vi "USRP Packet Transmitter(working).vi"(8 "Tx Parameters":T7={"Tx IQ Sampling\nRate [s/sec]"=500000.0, "Tx Frequency [Hz]"=2500000000.0, "Tx Gain [dB]"=0.0, "Tx Antenna"="TX1"} {"Tx Gain [dB]" format="%#.6p"; "Tx Frequency [Hz]" format="%#.6p"; "Tx IQ Sampling\nRate [s/sec]" format="%#.6p"}, 9 "USRP IP address":refnum<k15>="192.168.10.2", 10 "working directory":path=path "C:/perlTest") -> (1 "Constellation Graph":T1(graph), 2 "error out":errorcluster, 3 "standard output":string)   [LabVIEW 2022 SP3]
uses:
  <instrlib>/niUSRP/niUSRP Write Tx Data (CDB Cluster).vi
  <vilib>/addons/Modulation/Digital/General/MT Generate PSK System Parameters(M).vi
  <vilib>/addons/Modulation/niDMT.lvlib
panel:
  out "return value":string
  in  "module path":path
  out "error out 2":errorcluster
  in  "autoscale":bool
  out "Symbol Rate\n[symbols/sec]":dbl=25000.0 format="%#.6p"
  in  "stop":bool
  in  "Tab Control":T2(tab)
  in  "command line":string
  in  "Packet Parameters":T3={"Guard Bits "=30, "Sync Bits"=20, "Message Bits"=128}
  in  "Packet Pad \n[samples]":i32=200
  in  "Blank Frame \n[samples]":i32=500
  out "Number of Packets in Message":i32=46
  in  "PN sequence order\nfor Sync Bits":i32=31 caption="PN sequence order (9)"
  in  "Packet Repeat":i32=2
  in  "Select PSK Modulation Format":T4(tab)=enum."QPSK" caption="PSK"
  in  "BPSK System Parameters":T5={"Samples per Symbol"=8, "symbol map"=[], "Differential PSK"=enum."disable", "PSK type"=0} {"PSK type" items=["normal", "shifted", "offset"]; "symbol map" format="%.3f"}
  in  "QPSK System Parameters":T5={"Samples per Symbol"=8, "symbol map"=[], "Differential PSK"=enum."disable", "PSK type"=0} {"PSK type" items=["normal", "shifted", "offset"]; "symbol map" format="%.3f"}
  in  "pi/4 DQPSK System Parameters":T5={"Samples per Symbol"=8, "symbol map"=[], "Differential PSK"=enum."enable", "PSK type"=1} {"PSK type" items=["normal", "shifted", "offset"]; "symbol map" format="%.3f"}
  in  "OQPSK System Parameters":T5={"Samples per Symbol"=8, "symbol map"=[], "Differential PSK"=enum."disable", "PSK type"=2} {"PSK type" items=["normal", "shifted", "offset"]; "symbol map" format="%.3f"}
  in  "8-PSK System Parameters":T5={"Samples per Symbol"=8, "symbol map"=[], "Differential PSK"=enum."disable", "PSK type"=0} {"PSK type" items=["normal", "shifted", "offset"]; "symbol map" format="%.3f"}
  in  "16-PSK System Parameters":T5={"Samples per Symbol"=8, "symbol map"=[], "Differential PSK"=enum."disable", "PSK type"=0} {"PSK type" items=["normal", "shifted", "offset"]; "symbol map" format="%.3f"}
  in  "M":i32=4 min=2 step=2
  in  "Custom System Parameters":T5={"Samples per Symbol"=8, "symbol map"=[], "Differential PSK"=enum."disable", "PSK type"=0} {"PSK type" items=["normal", "shifted", "offset"]; "symbol map" format="%.3f"}
  in  "Pulse Shaping Filter Parameters":T6={"Alpha"=0.5, "Filter Length"=6, "TX Filter"=enum."Root Raised Cos"} caption="Pulse Shaping Filter" {"Alpha" format="%.2f"}
  out "Actual Tx Parameters":T7={"Tx IQ Sampling\nRate [s/sec]"=200000.0, "Tx Frequency [Hz]"=2500000000.0, "Tx Gain [dB]"=0.0, "Tx Antenna"="TX1"} {"Tx Gain [dB]" format="%#.6p"; "Tx Frequency [Hz]" format="%#.6p"; "Tx IQ Sampling\nRate [s/sec]" format="%#.6p"}
  in  "Queue Length":i32=10
  # "Packet Transmitter"
  # "Guard\nBand"
  # "Sync\nSeq"
  # "Packet\nNumber"
  # "Pad\nData"
  # "Blank\nFrame"
  # "Data"
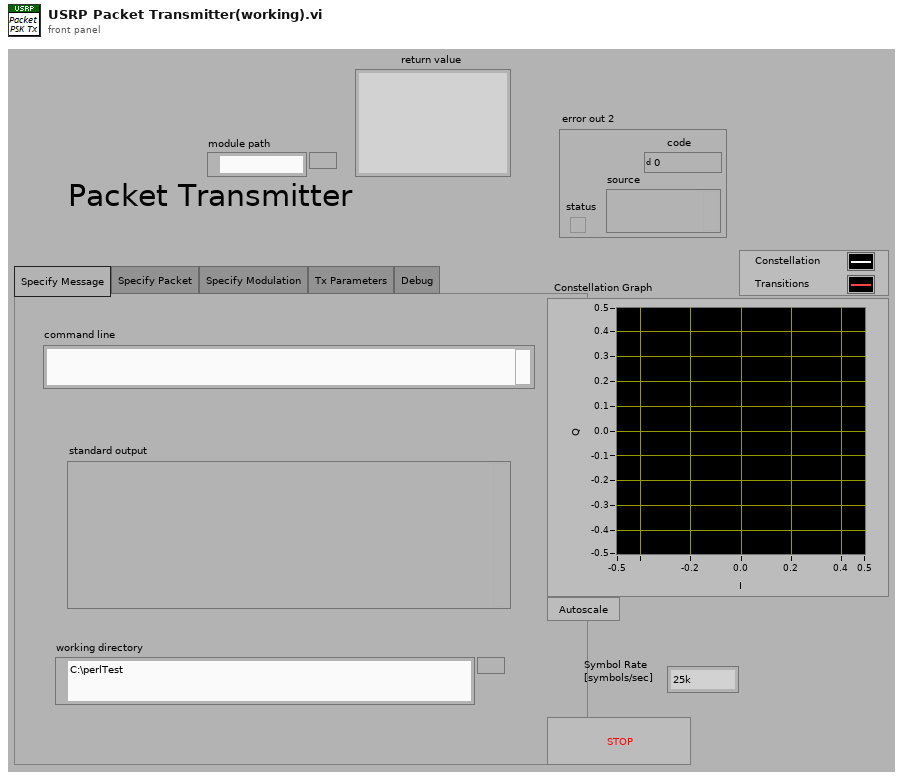
[diagram p1: front panel]
types:
  T1 = cluster{"Decimated Array":dbl[], "Decimated Array":dbl[]}[]
  T2 = enum32{"Specify Message", "Specify Packet", "Specify Modulation", "Tx Parameters", "Debug"}
  T3 = cluster{"Guard Bits ":i32, "Sync Bits":i32, "Message Bits":i32}
  T4 = enum32{"BPSK", "QPSK", "pi/4DQPSK", "OQPSK", "8-PSK", "16-PSK", "Custom"}
  T5 = cluster{"Samples per Symbol":i32, "symbol map":cdb[], "Differential PSK":enum16{"disable", "enable"}, "PSK type":u16}
  T6 = cluster{"Alpha":dbl, "Filter Length":i32, "TX Filter":enum16{"none", "Raised Cosine", "Root Raised Cos", "Gaussian"}}
  T7 = cluster{"Tx IQ Sampling\nRate [s/sec]":dbl, "Tx Frequency [Hz]":dbl, "Tx Gain [dB]":dbl, "Tx Antenna":string}
  T8 = cluster{"samples per symbol (16)":i32, "symbol map":cdb[], "differential PSK":enum16{"disable", "enable"}, "PSK type":u16}
  T9 = cluster{"s? t:f":cluster{"t0":dbl, "dt":dbl, "Y":cdb[]}, i32}
  T10 = cluster{"output complex waveform":cluster{"t0":dbl, "dt":dbl, "Y":cdb[]}, i32}
  T11 = cluster{"constellation":dbl[], "oversampled data":dbl[]}[]
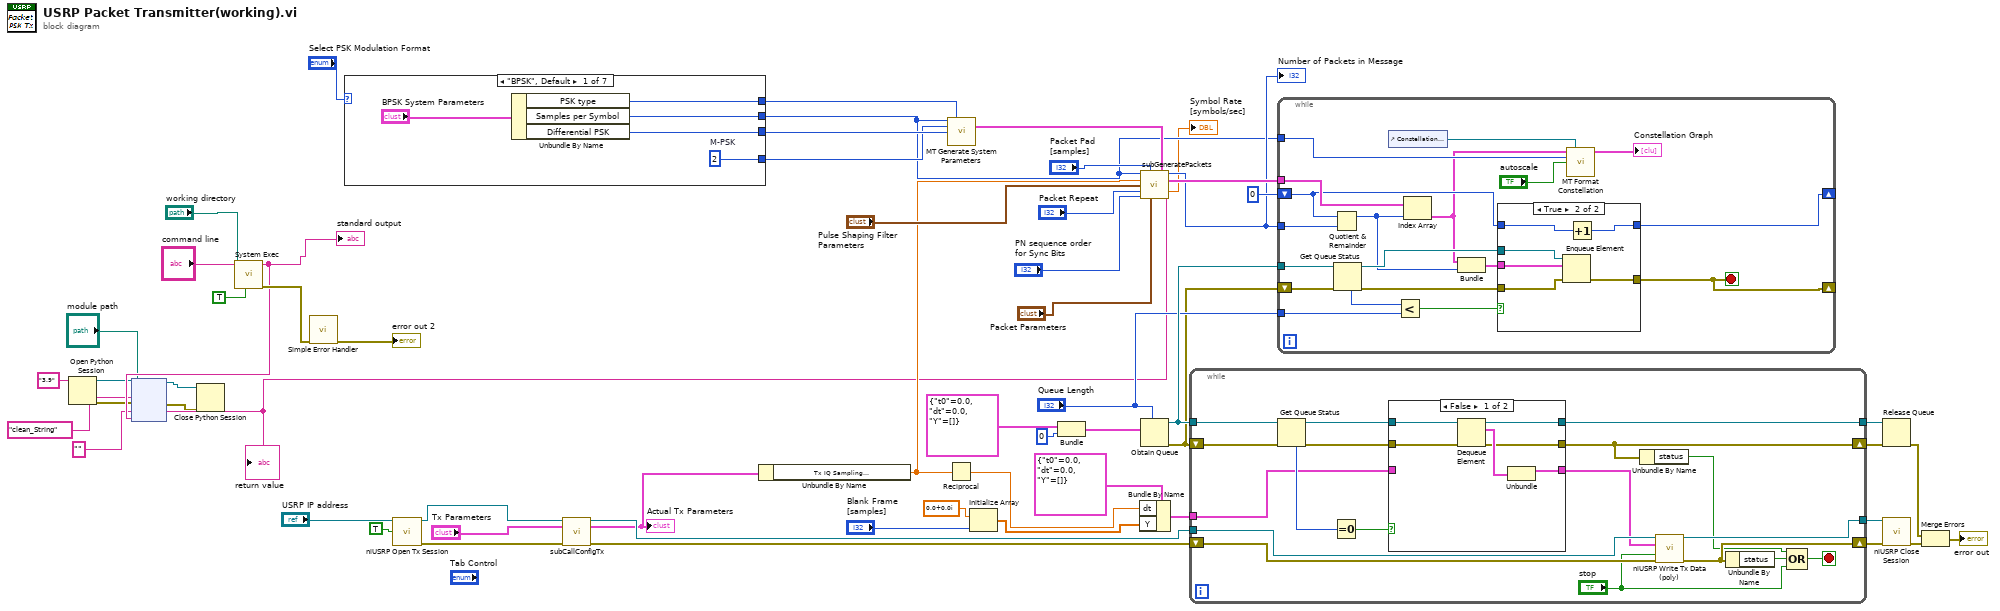
[diagram p0: block diagram]
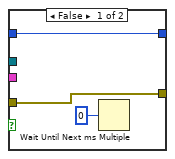
[diagram p2: hidden frame]
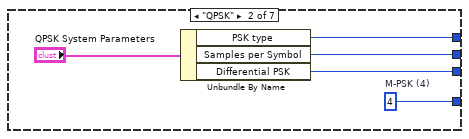
[diagram p3: hidden frame]
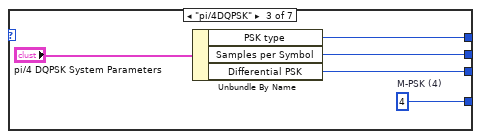
[diagram p4: hidden frame]
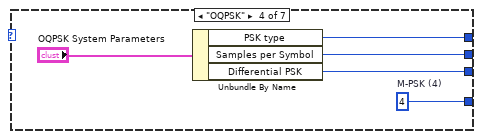
[diagram p5: hidden frame]
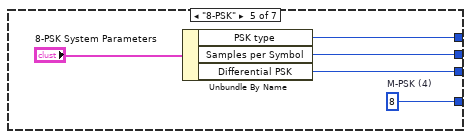
[diagram p6: hidden frame]
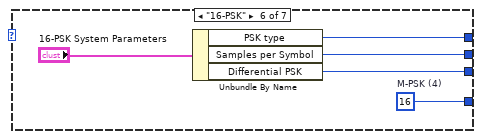
[diagram p7: hidden frame]
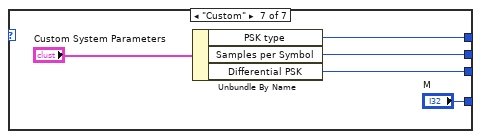
[diagram p8: hidden frame]
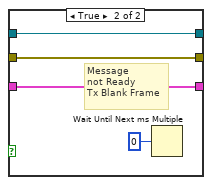
[diagram p9: hidden frame]
diagram:
  n1 = Open Python Session(python version="3.9" ("Python version")) -> (session out=w7:refnum<k35>, error out=w6:errorcluster)  [unwired: 2 in]
  n2 = call <vilib>:"System Exec.vi"("run minimized? (F)"=TRUE, "working directory"="working directory", "command line"="command line") -> ("error out"=w13:errorcluster, "standard output"=w10:string)  [unwired: 3 in, 4 out]
  "standard output" <- w10
  n3 = node(w7, "module path", "clean_String" ("function name"), w6, "", w10) -> (w5:refnum<k35>, w4:errorcluster, w9:string)  [unwired: 1 in, 2 out]
  "return value" <- w9
  n4 = Close Python Session(session in=w5, error in=w4) -> ()  [unwired: 1 out]
  n5 = call <vilib>:"Simple Error Handler.vi"("error in (no error)"=w13) -> ("error out"=→"error out 2":errorcluster)  [unwired: 1 in, 7 out]
  n6 = case shown="\"BPSK\", Default" "Select PSK Modulation Format" {
    tunnel: [w60 w64 w72 w77 w82 w88 w91] -> w17
    tunnel: [w61 w66 w71 w76 w81 w87 w92] -> w56
    tunnel: [w63 w68 w73 w78 w80 w86 "M"] -> w38
    tunnel: [w62 w67 w70 w75 w83 w85 w93] -> w25
    frame "BPSK", Default {
      w63 = 2  # M-PSK
      n7 = Unbundle By Name("BPSK System Parameters") -> ("PSK type"=w62:u16, "Samples per Symbol"=w60:i32, "Differential PSK"=w61:enum16{"disable", "enable"})
    }
    frame "QPSK" {
      w68 = 4  # M-PSK (4)
      n8 = Unbundle By Name("QPSK System Parameters") -> ("PSK type"=w67:u16, "Samples per Symbol"=w64:i32, "Differential PSK"=w66:enum16{"disable", "enable"})
    }
    frame "pi/4DQPSK" {
      w73 = 4  # M-PSK (4)
      n9 = Unbundle By Name("pi/4 DQPSK System Parameters") -> ("PSK type"=w70:u16, "Samples per Symbol"=w72:i32, "Differential PSK"=w71:enum16{"disable", "enable"})
    }
    frame "OQPSK" {
      w78 = 4  # M-PSK (4)
      n10 = Unbundle By Name("OQPSK System Parameters") -> ("PSK type"=w75:u16, "Samples per Symbol"=w77:i32, "Differential PSK"=w76:enum16{"disable", "enable"})
    }
    frame "8-PSK" {
      w80 = 8  # M-PSK (4)
      n11 = Unbundle By Name("8-PSK System Parameters") -> ("PSK type"=w83:u16, "Samples per Symbol"=w82:i32, "Differential PSK"=w81:enum16{"disable", "enable"})
    }
    frame "16-PSK" {
      w86 = 16  # M-PSK (4)
      n12 = Unbundle By Name("16-PSK System Parameters") -> ("PSK type"=w85:u16, "Samples per Symbol"=w88:i32, "Differential PSK"=w87:enum16{"disable", "enable"})
    }
    frame "Custom" {
      n13 = Unbundle By Name("Custom System Parameters") -> ("PSK type"=w93:u16, "Samples per Symbol"=w91:i32, "Differential PSK"=w92:enum16{"disable", "enable"})
    }
  }
  n14 = call <instrlib>:"niUSRP Open Tx Session.vi"("device names"="USRP IP address", "reset"=TRUE) -> ("session handle out"=w29:refnum<k15>, "error out"=w28:errorcluster)  [unwired: 12 in]
  n15 = call "subCallConfigTx.vi"("session handle"=w29, "Tx Parameters"="Tx Parameters", "error in"=w28) -> ("session handle out"=w37:refnum<k15>, "Actual Tx Parameters"=w36:T7, "error out"=w42:errorcluster)  [unwired: 10 in]
  "Actual Tx Parameters" <- w36
  n16 = Unbundle By Name(w36) -> ("Tx IQ Sampling\nRate [s/sec]"=w18:dbl)
  n17 = call-poly <vilib>:"MT Generate System Parameters.vi"("samples per symbol (16)"=w17, "PSK type"=w25, "M-PSK (4)"=w38, "differential PSK"=w56) -> ("PSK system parameters"=w26:T8)  [unwired: 9 in, 2 out]
  n18 = Reciprocal(x=w18) -> (1/x=w39:dbl)
  n19 = Initialize Array(cdb 0.0+0.0i ("element"), "Blank Frame \n[samples]") -> (w52:cdb[])
  n20 = Bundle("s? t:f"=cluster{"t0":dbl, "dt":dbl, "Y":cdb[]} {"t0"=0.0, "dt"=0.0, "Y"=[]}, 0) -> (w47:T9)  [unwired: 1 in]
  n21 = Bundle By Name(cluster=cluster{"t0":dbl, "dt":dbl, "Y":cdb[]} {"t0"=0.0, "dt"=0.0, "Y"=[]} ("s? t:f"), "dt"=w39, "Y"=w52) -> (w51:cluster{"t0":dbl, "dt":dbl, "Y":cdb[]})
  n22 = call "subGeneratePackets.vi"("Samples per Symbol"=w17, "Packet Pad \n[samples]"="Packet Pad \n[samples]", "PSK system parameters"=w26, "Tx IQ Sampling\nRate [s/sec]"=w18, "Pulse Shaping Filter Parameters"="Pulse Shaping Filter Parameters", "Packet Repeat"="Packet Repeat", "PN sequence order\nfor Sync Bits"="PN sequence order\nfor Sync Bits", "Packet Parameters"="Packet Parameters", "Message Text"=w9) -> ("Number of Packets"=w35:i32, "Packets"=w44:cluster{"t0":dbl, "dt":dbl, "Y":cdb[]}[], "Symbol Rate"=→"Symbol Rate\n[symbols/sec]":dbl)  [unwired: 4 in]
  "Number of Packets in Message" <- w35
  n23 = Obtain Queue(max queue size (-1, unlimited)="Queue Length", element data type=w47) -> (queue out=w53:refnum<queue>, error out=w31:errorcluster)  [unwired: 3 in, 1 out]
  n24 = while {
    tunnel: w37 -> [w102]
    shift-right: [w99] -> w41
    shift-left: w42 -> [w103]
    tunnel: w53 -> [w111]
    tunnel: w51 -> [w108]
    tunnel: [w107] -> w50
    tunnel: [w101] -> w40
    shift-right: [w96] -> w49
    shift-left: w31 -> [w104]
    stop <- w98 stop-if-true
    n25 = Get Queue Status(queue=w111, error in (no error)=w104) -> (queue out=w106:refnum<queue>, error out=w105:errorcluster, # elements in queue=w110:i32)  [unwired: 1 in, 5 out]
    n26 = Equal To 0?(x=w110) -> (x = 0?=w109:bool)
    n27 = case shown="False" w109 {
      tunnel: w108 -> [_ w121]
      tunnel: [w113 w121] -> w94
      tunnel: [w117 w119] -> w107
      tunnel: [w112 w120] -> w96
      tunnel: w106 -> [w116 w119]
      tunnel: w105 -> [w115 w120]
      frame False {
        n28 = Dequeue Element(queue=w116, error in (no error)=w115) -> (queue out=w117:refnum<queue>, element=w114:T9, error out=w112:errorcluster)  [unwired: 1 in, 1 out]
        n29 = Unbundle(w114) -> ("s? t:f"=w113:cluster{"t0":dbl, "dt":dbl, "Y":cdb[]})  [unwired: 1 out]
      }
      frame True {
        # "Message\nnot Ready\nTx Blank Frame"
        n30 = Wait Until Next ms Multiple(millisecond multiple=u32 0) -> ()  [unwired: 1 out]
      }
    }
    n31 = Unbundle By Name(w96) -> ("status"=w95:bool)
    n32 = call-poly <instrlib>:"niUSRP Write Tx Data (poly).vi"("session handle"=w102, "data"=w94, "end of data?"="stop", "error in (no error)"=w103) -> ("session handle out"=w101:refnum<k15>, "error out"=w99:errorcluster)  [unwired: 10 in]
    n33 = Unbundle By Name(w99) -> ("status"=w100:bool)
    n34 = Compound Arithmetic op=OR(w95, w100, "stop") -> (w98:bool)
  }
  n35 = while {
    tunnel: w53 -> [w140]
    shift-right: [w133] -> _
    shift-left: 0 -> [w129]
    tunnel: w44 -> [w130]
    tunnel: "Queue Length" -> [w132]
    tunnel: w35 -> [w131]
    shift-right: [w127] -> _
    shift-left: w31 -> [w135]
    tunnel: w17 -> [w124]
    stop <- w127 stop-if-true
    n36 = Quotient & Remainder(x=w129, y=w131) -> (x-y*floor(x/y)=w128:i32)  [unwired: 1 out]
    n37 = Get Queue Status(queue=w140, error in (no error)=w135) -> (queue out=w139:refnum<queue>, error out=w136:errorcluster, # elements in queue=w138:i32)  [unwired: 1 in, 5 out]
    n38 = control-ref of="Constellation Graph"() -> (w125:refnum<vi>)
    n39 = Less?(x=w138, y=w132) -> (x < y?=w137:bool)
    n40 = Index Array(array=w130, index=w128) -> (element=w122:cluster{"t0":dbl, "dt":dbl, "Y":cdb[]})
    n41 = Bundle("output complex waveform"=w122, w128) -> (w134:T10)  [unwired: 1 in]
    n42 = case shown="True" w137 {
      tunnel: w136 -> [w141 w149]
      tunnel: w139 -> [_ w148]
      tunnel: [w141 w147] -> w127
      tunnel: w134 -> [_ w146]
      tunnel: w129 -> [w143 w145]
      tunnel: [w143 w144] -> w133
      frame False {
        n43 = Wait Until Next ms Multiple(millisecond multiple=u32 0) -> ()  [unwired: 1 out]
      }
      frame True {
        n44 = Enqueue Element(queue=w148, element=w146, error in (no error)=w149) -> (error out=w147:errorcluster)  [unwired: 1 in, 2 out]
        n45 = Increment(x=w145) -> (x+1=w144:i32)
      }
    }
    n46 = call <vilib>:"MT Format Constellation.vi"("waveform"=w122, "constellation reference"=w125, "samples per symbol"=w124, "autoscale"="autoscale") -> ("constellation graph"=→"Constellation Graph":T11)  [unwired: 1 in, 10 out]
  }
  n47 = Release Queue(queue=w50, error in (no error)=w49) -> (error out=w24:errorcluster)  [unwired: 3 out]
  n48 = call <instrlib>:"niUSRP Close Session.vi"("session handle"=w40, "error in (no error)"=w41) -> ("error out"=w23:errorcluster)  [unwired: 13 in]
  n49 = Merge Errors(w24, w23) -> (→"error out":errorcluster)
